vi "IDN.vi"(8 "error in (no error)":errorcluster, 11 "VISA resource name":refnum<visa-resource-name>) -> (0 "error out":errorcluster, 1 "Serial Number":string, 2 "Model":string, 3 "VISA Refnum out":refnum<visa-resource-name>, 4 "Firmware (Major.Minor.Release)":string, 5 "Manufacturer":string)   [LabVIEW 2019, in "RP100.lvlib"]
uses:
  RP100.lvlib
panel:
  out "*IDN?":string
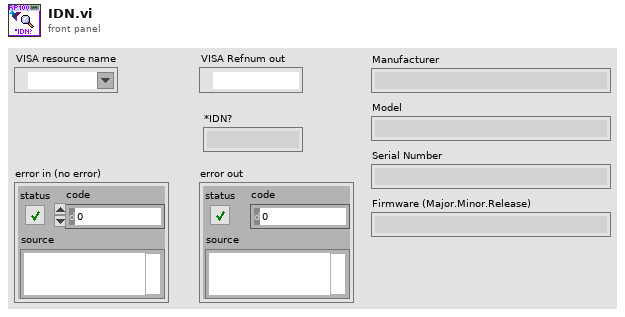
[diagram p1: front panel]
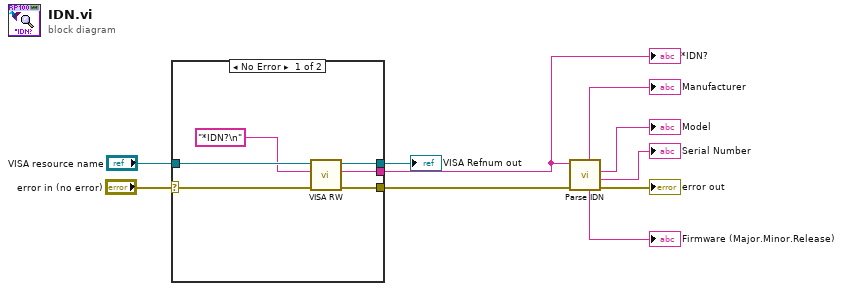
[diagram p0: block diagram]
diagram:
  n1 = case shown="No Error" "error in (no error)" {
    selector: "error in (no error)" -> [w13 w18]
    tunnel: [w16 w17] -> w10
    tunnel: "VISA resource name" -> [w15 w17]
    tunnel: [w14 w18] -> w6
    tunnel: [w12 _] -> w2
    frame No Error {
      n2 = call "VISA RW.vi"("error in (no error)"=w13, "Write"="*IDN?\n" ("format string"), "VISA Refnum in"=w15) -> ("error out"=w14:errorcluster, "Read"=w12:string, "VISA Refnum out"=w16:refnum<visa-resource-name>)  [unwired: 6 in]
    }
    frame Error {
    }
  }
  "*IDN?" <- w2
  "VISA Refnum out" <- w10
  n3 = call "Parse IDN.vi"("error in (no error)"=w6, "*IDN?"=w2) -> ("error out"=→"error out":errorcluster, "Serial Number"=→"Serial Number":string, "Model"=→"Model":string, "Firmware (Major.Minor.Release)"=→"Firmware (Major.Minor.Release)":string, "Manufacturer"=→"Manufacturer":string)  [unwired: 5 in]
